vi "get Tests.vi"(8 "error in (no error)":errorcluster, 11 "Norm in":refnum<class "Norm.lvclass">) -> (0 "error out":errorcluster, 2 "Tests":refnum<class "Test.lvclass">[](array[class]), 3 "Norm out":refnum<class "Norm.lvclass">)   [LabVIEW 2013, in "DatenKlassen.lvlib" / "Norm.lvclass"]
uses:
  Norm.lvclass
  Test/Test.lvclass
  Norm.lvclass/Norm.ctl
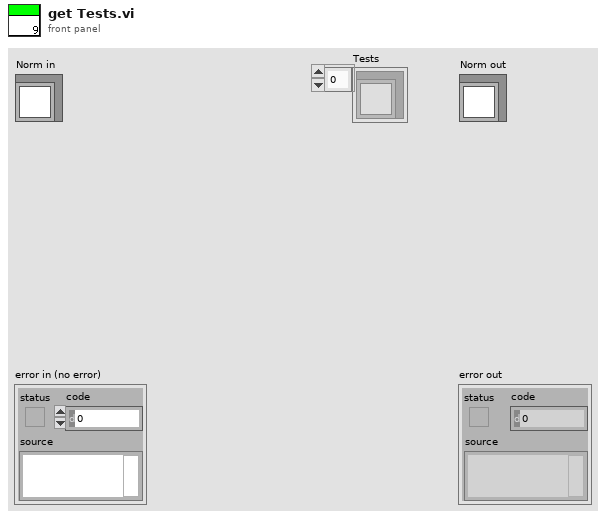
[diagram p1: front panel]
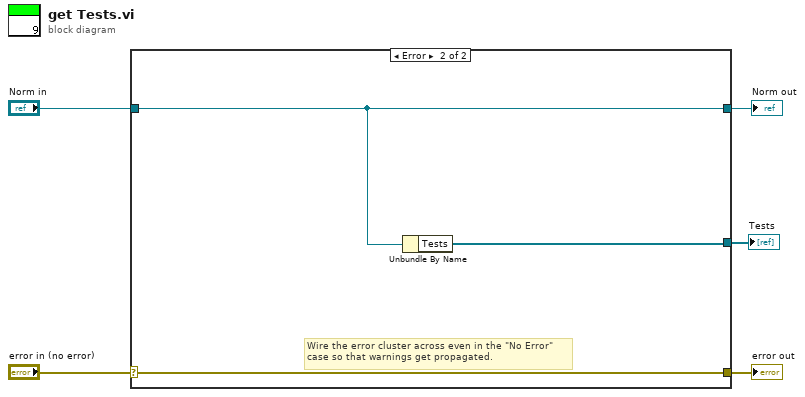
[diagram p0: block diagram]
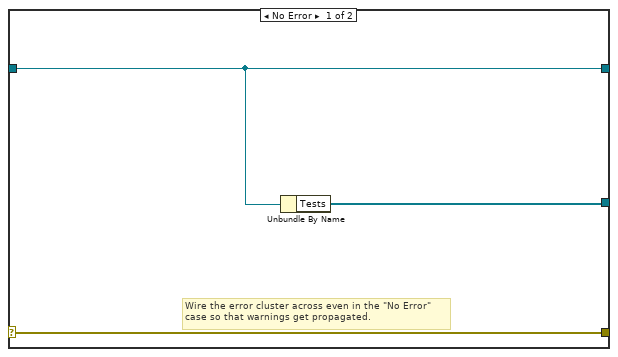
[diagram p2: hidden frame]
diagram:
  n1 = case shown="Error" "error in (no error)" {
    selector: "error in (no error)" -> [w8 w11]
    tunnel: [w8 w11] -> w4
    tunnel: [w7 w10] -> w2
    tunnel: "Norm in" -> [w7 w10]
    tunnel: [w6 w9] -> w1
    frame No Error {
      # "Wire the error cluster across even in the \"No Error\"\ncase so that warnings get propagated."
      n2 = Unbundle By Name(w7) -> ("Tests"=w6:refnum<class "Test.lvclass">[])
    }
    frame Error {
      # "Wire the error cluster across even in the \"No Error\"\ncase so that warnings get propagated."
      n3 = Unbundle By Name(w10) -> ("Tests"=w9:refnum<class "Test.lvclass">[])
    }
  }
  "error out" <- w4
  "Norm out" <- w2
  "Tests" <- w1
